vi "Refnum Initialize.vi"(8 "error in (no error)":errorcluster, 11 "QMenu Class in":refnum<class "QMenu Class.lvclass">) -> (0 "error out":errorcluster, 3 "QMenu Class out":refnum<class "QMenu Class.lvclass">)   [LabVIEW 2020, in "QTab.lvlib" / "QMenu Class.lvclass"]
uses:
  QMenu Class.lvclass
  Command Data.ctl
  Command.ctl
  Active Event Data.ctl
  Close Event Data.ctl
  Drag Event Data.ctl
  Image Data.ctl
  <vilib>/picture/picture.llb/imagedata.ctl
  Button Attribute.ctl
  Parameter.ctl
  QMenu Class.lvclass/QMenu Class.ctl
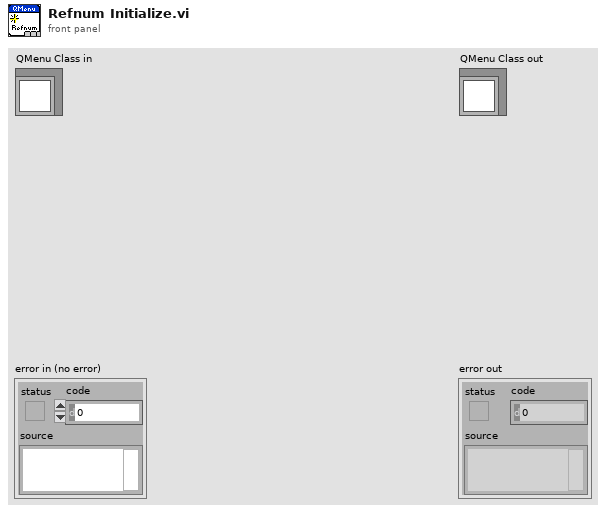
[diagram p1: front panel]
types:
  T1 = typedef "QTab.lvlib/QMenu Class.lvclass/Parameter.ctl" = cluster{"Close Timeout":i32, "Drag Timeout":i32}
  T2 = typedef "QTab.lvlib/QMenu Class.lvclass/Button Attribute.ctl" = cluster{"Label":string, "Button Text":string, "Closable":bool, "Draggable":bool}
  T3 = typedef "QTab.lvlib/QMenu Class.lvclass/Image Data.ctl" = cluster{"Button Image":T4, "Close Button Image":T4, "Left Button Image":T4, "Right Button Image":T4}
  T4 = typedef "imagedata.ctl" = cluster{"image type":i32, "image depth":i32, "image":u8[], "mask":u8[], "colors":u32[], "Rectangle":cluster{"left":i16, "top":i16, "right":i16, "bottom":i16}}
  T5 = typedef "QTab.lvlib/QMenu Class.lvclass/Drag Event Data.ctl" = cluster{"Index":i32, "Label":string, "Vertical":i32, "Horizontal":i32, "Confirm Notifier":refnum<notifier>}
  T6 = typedef "QTab.lvlib/QMenu Class.lvclass/Close Event Data.ctl" = cluster{"Index":i32, "Label":string, "Confirm Notifier":refnum<notifier>}
  T7 = typedef "QTab.lvlib/QMenu Class.lvclass/Active Event Data.ctl" = cluster{"Index":i32, "Label":string}
  T8 = typedef "QTab.lvlib/QMenu Class.lvclass/Command Data.ctl" = cluster{"Command":T9, "Data":variant}
  T9 = typedef "QTab.lvlib/QMenu Class.lvclass/Command.ctl" = enum16{"Initialize", "Get Active Button", "Set Active Button", "Set Button Attribute", "Add Button", "Close Button", "Draw", "Stop"}
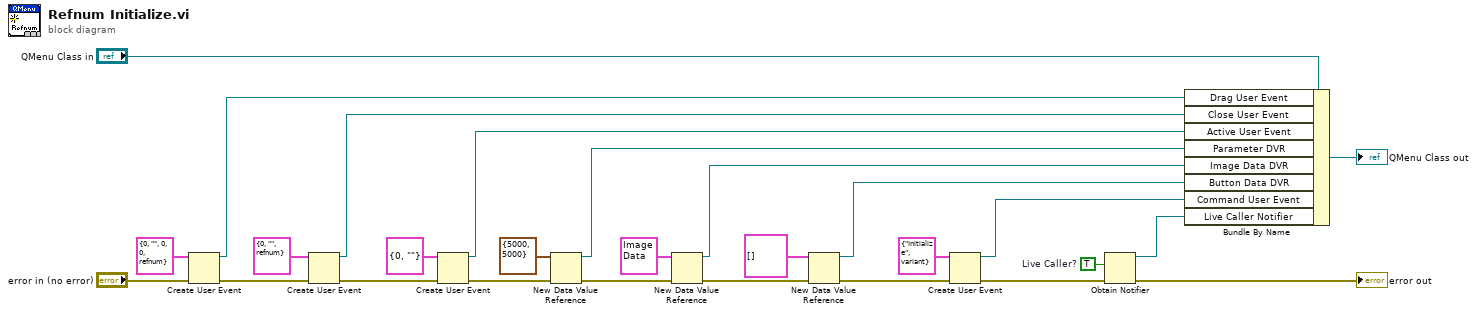
[diagram p0: block diagram]
diagram:
  w23 = TRUE  # Live Caller?
  n1 = Create User Event(user event datatype=T5 {"Index"=0, "Label"="", "Vertical"=0, "Horizontal"=0, "Confirm Notifier"=refnum} ("Drag Event Data"), error in="error in (no error)") -> (user event=w8:refnum<user-event>, error out=w11:errorcluster)
  n2 = Create User Event(user event datatype=T6 {"Index"=0, "Label"="", "Confirm Notifier"=refnum} ("Close Event Data"), error in=w11) -> (user event=w12:refnum<user-event>, error out=w13:errorcluster)
  n3 = Create User Event(user event datatype=T7 {"Index"=0, "Label"=""} ("Active Event Data"), error in=w13) -> (user event=w15:refnum<user-event>, error out=w4:errorcluster)
  n4 = New Data Value Reference(data value=T1 {"Close Timeout"=5000, "Drag Timeout"=5000} ("Parameter"), error in=w4) -> (data value reference=w1:refnum<data-value>, error out=w2:errorcluster)
  n5 = New Data Value Reference(data value=T3 {"Button Image"={"image type"=0, "image depth"=24, "image"=array[19200 elements], "mask"=[], "colors"=[], "Rectangle"={"left"=0, "top"=0, "right"=200, "bottom"=32}}, "Close Button Image"={"image type"=0, "image depth"=32, "image"=[0, 0, 0, 0, 0, 0, 0, 0, 0, 0, 0, 0, 0, 0, 0, 0, 0, 0, 0, 0, 0, 0, 0, 0, 0, 0, 0, 0, 0, 0, 0, 0, 0, 0, 0, 0, 0, 0, 0, 0, 0, 0, 0, 0, 0, 0, 0, 0, 0, 0, 0, 0, 0, 0, 0, 0, 0, 0, 0, 0, 0, 0, 0, 0, 0, 0, 0, 0, 0, 0, 0, 0, 0, 0, 0, 0, 0, 0, 0, 0, 0, 0, 0, 0, 0, 0, 0, 0, 0, 0, 0, 0, 0, 0, 0, 0, 0, 0, 0, 0, 0, 0, 0, 0, 0, 0, 0, 0, 0, 0, 0, 0, 0, 0, 0, 0, 0, 0, 0, 0, 0, 0, 0, 0, 0, 0, 0, 0, 0, 0, 0, 0, 0, 0, 0, 0, 0, 0, 0, 0, 0, 0, 0, 0, 0, 0, 0, 0, 0, 0, 0, 0, 42, 152, 164, 164, 175, 149, 165, 166, 187, 149, 165, 166, 187, 149, 165, 166, 187, 149, 165, 166, 187, 149, 165, 166, 187, 149, 165, 166, 187, 149, 165, 166, 187, 149, 165, 166, 187, 149, 165, 166, 187, 149, 165, 166, 187, 149, 165, 166, 175, 149, 165, 166, 41, 149, 168, 168, 0, 0, 0, 0, 0, 0, 0, 0, 0, 0, 0, 0, 0, 0, 0, 0, 176, 149, 165, 167, 238, 149, 165, 166, 187, 149, 165, 166, 187, 149, 165, 166, 187, 149, 165, 166, 187, 149, 165, 166, 187, 149, 165, 166, 187, 149, 165, 166, 187, 149, 165, 166, 187, 149, 165, 166, 187, 149, 165, 166, 187, 149, 165, 166, 238, 149, 165, 166, 175, 149, 165, 166, 0, 0, 0, 0, 0, 0, 0, 0, 0, 0, 0, 0, 0, 0, 0, 0, 191, 150, 166, 166, 191, 150, 166, 166, 0, 0, 0, 0, 0, 0, 0, 0, 0, 0, 0, 0, 0, 0, 0, 0, 0, 0, 0, 0, 0, 0, 0, 0, 0, 0, 0, 0, 0, 0, 0, 0, 0, 0, 0, 0, 0, 0, 0, 0, 191, 150, 166, 166, 191, 150, 166, 166, 0, 0, 0, 0, 0, 0, 0, 0, 0, 0, 0, 0, 0, 0, 0, 0, 191, 150, 166, 166, 191, 150, 166, 166, 0, 0, 0, 0, 25, 153, 163, 163, 118, 149, 164, 166, 0, 0, 0, 0, 0, 0, 0, 0, 0, 0, 0, 0, 0, 0, 0, 0, 118, 149, 164, 166, 25, 153, 163, 163, 0, 0, 0, 0, 191, 150, 166, 166, 191, 150, 166, 166, 0, 0, 0, 0, 0, 0, 0, 0, 0, 0, 0, 0, 0, 0, 0, 0, 191, 150, 166, 166, 191, 150, 166, 166, 0, 0, 0, 0, 119, 150, 165, 165, 255, 149, 165, 166, 142, 149, 165, 165, 0, 0, 0, 0, 0, 0, 0, 0, 142, 149, 165, 165, 255, 149, 165, 166, 119, 150, 165, 165, 0, 0, 0, 0, 191, 150, 166, 166, 191, 150, 166, 166, 0, 0, 0, 0, 0, 0, 0, 0, 0, 0, 0, 0, 0, 0, 0, 0, 191, 150, 166, 166, 191, 150, 166, 166, 0, 0, 0, 0, 0, 0, 0, 0, 142, 149, 165, 165, 255, 149, 165, 166, 142, 149, 165, 165, 142, 149, 165, 165, 255, 149, 165, 166, 142, 149, 165, 165, 0, 0, 0, 0, 0, 0, 0, 0, 191, 150, 166, 166, 191, 150, 166, 166, 0, 0, 0, 0, 0, 0, 0, 0, 0, 0, 0, 0, 0, 0, 0, 0, 191, 150, 166, 166, 191, 150, 166, 166, 0, 0, 0, 0, 0, 0, 0, 0, 0, 0, 0, 0, 135, 149, 164, 166, 255, 149, 165, 166, 255, 149, 165, 166, 143, 150, 166, 166, 0, 0, 0, 0, 0, 0, 0, 0, 0, 0, 0, 0, 191, 150, 166, 166, 191, 150, 166, 166, 0, 0, 0, 0, 0, 0, 0, 0, 0, 0, 0, 0, 0, 0, 0, 0, 191, 150, 166, 166, 191, 150, 166, 166, 0, 0, 0, 0, 0, 0, 0, 0, 0, 0, 0, 0, 135, 149, 164, 166, 255, 149, 165, 166, 255, 149, 165, 166, 143, 150, 166, 166, 0, 0, 0, 0, 0, 0, 0, 0, 0, 0, 0, 0, 191, 150, 166, 166, 191, 150, 166, 166, 0, 0, 0, 0, 0, 0, 0, 0, 0, 0, 0, 0, 0, 0, 0, 0, 191, 150, 166, 166, 191, 150, 166, 166, 0, 0, 0, 0, 0, 0, 0, 0, 142, 149, 165, 165, 255, 149, 165, 166, 142, 149, 165, 165, 142, 149, 165, 165, 255, 149, 165, 166, 142, 149, 165, 165, 0, 0, 0, 0, 0, 0, 0, 0, 191, 150, 166, 166, 191, 150, 166, 166, 0, 0, 0, 0, 0, 0, 0, 0, 0, 0, 0, 0, 0, 0, 0, 0, 191, 150, 166, 166, 191, 150, 166, 166, 0, 0, 0, 0, 119, 150, 165, 165, 255, 149, 165, 166, 142, 149, 165, 165, 0, 0, 0, 0, 0, 0, 0, 0, 142, 149, 165, 165, 255, 149, 165, 166, 119, 150, 165, 165, 0, 0, 0, 0, 191, 150, 166, 166, 191, 150, 166, 166, 0, 0, 0, 0, 0, 0, 0, 0, 0, 0, 0, 0, 0, 0, 0, 0, 191, 150, 166, 166, 191, 150, 166, 166, 0, 0, 0, 0, 25, 153, 163, 163, 118, 149, 164, 166, 0, 0, 0, 0, 0, 0, 0, 0, 0, 0, 0, 0, 0, 0, 0, 0, 118, 149, 164, 166, 25, 153, 163, 163, 0, 0, 0, 0, 191, 150, 166, 166, 191, 150, 166, 166, 0, 0, 0, 0, 0, 0, 0, 0, 0, 0, 0, 0, 0, 0, 0, 0, 191, 150, 166, 166, 191, 150, 166, 166, 0, 0, 0, 0, 0, 0, 0, 0, 0, 0, 0, 0, 0, 0, 0, 0, 0, 0, 0, 0, 0, 0, 0, 0, 0, 0, 0, 0, 0, 0, 0, 0, 0, 0, 0, 0, 0, 0, 0, 0, 191, 150, 166, 166, 191, 150, 166, 166, 0, 0, 0, 0, 0, 0, 0, 0, 0, 0, 0, 0, 0, 0, 0, 0, 176, 149, 165, 167, 238, 149, 165, 166, 187, 149, 165, 166, 187, 149, 165, 166, 187, 149, 165, 166, 187, 149, 165, 166, 187, 149, 165, 166, 187, 149, 165, 166, 187, 149, 165, 166, 187, 149, 165, 166, 187, 149, 165, 166, 187, 149, 165, 166, 238, 149, 165, 166, 175, 149, 165, 166, 0, 0, 0, 0, 0, 0, 0, 0, 0, 0, 0, 0, 0, 0, 0, 0, 41, 149, 168, 168, 174, 149, 166, 166, 187, 149, 165, 166, 187, 149, 165, 166, 187, 149, 165, 166, 187, 149, 165, 166, 187, 149, 165, 166, 187, 149, 165, 166, 187, 149, 165, 166, 187, 149, 165, 166, 187, 149, 165, 166, 187, 149, 165, 166, 174, 149, 166, 166, 41, 149, 168, 168, 0, 0, 0, 0, 0, 0, 0, 0, 0, 0, 0, 0, 0, 0, 0, 0, 0, 0, 0, 0, 0, 0, 0, 0, 0, 0, 0, 0, 0, 0, 0, 0, 0, 0, 0, 0, 0, 0, 0, 0, 0, 0, 0, 0, 0, 0, 0, 0, 0, 0, 0, 0, 0, 0, 0, 0, 0, 0, 0, 0, 0, 0, 0, 0, 0, 0, 0, 0, 0, 0, 0, 0, 0, 0, 0, 0, 0, 0, 0, 0, 0, 0, 0, 0, 0, 0, 0, 0, 0, 0, 0, 0, 0, 0, 0, 0, 0, 0, 0, 0, 0, 0, 0, 0, 0, 0, 0, 0, 0, 0, 0, 0, 0, 0, 0, 0, 0, 0, 0, 0, 0, 0, 0, 0, 0, 0, 0, 0, 0, 0, 0, 0, 0, 0, 0, 0, 0, 0, 0, 0, 0, 0, 0, 0, 0, 0, 0, 0, 0, 0, 0, 0], "mask"=[0, 0, 0, 0, 0, 0, 0, 0, 31, 254, 0, 0, 63, 255, 0, 0, 48, 3, 0, 0, 48, 3, 0, 0, 51, 51, 0, 0, 51, 243, 0, 0, 49, 227, 0, 0, 49, 227, 0, 0, 51, 243, 0, 0, 51, 51, 0, 0, 48, 3, 0, 0, 48, 3, 0, 0, 63, 255, 0, 0, 31, 254, 0, 0, 0, 0, 0, 0, 0, 0, 0, 0], "colors"=[], "Rectangle"={"left"=0, "top"=0, "right"=18, "bottom"=18}}, "Left Button Image"={"image type"=0, "image depth"=32, "image"=array[2304 elements], "mask"=[0, 0, 0, 0, 0, 0, 0, 0, 0, 0, 0, 0, 15, 255, 240, 0, 31, 255, 248, 0, 24, 0, 24, 0, 24, 0, 24, 0, 24, 4, 24, 0, 24, 14, 24, 0, 24, 28, 24, 0, 24, 56, 24, 0, 24, 112, 24, 0, 24, 112, 24, 0, 24, 56, 24, 0, 24, 28, 24, 0, 24, 14, 24, 0, 24, 4, 24, 0, 24, 0, 24, 0, 24, 0, 24, 0, 31, 255, 248, 0, 15, 255, 240, 0, 0, 0, 0, 0, 0, 0, 0, 0, 0, 0, 0, 0], "colors"=[], "Rectangle"={"left"=0, "top"=4, "right"=24, "bottom"=28}}, "Right Button Image"={"image type"=0, "image depth"=32, "image"=array[2304 elements], "mask"=[0, 0, 0, 0, 0, 0, 0, 0, 0, 0, 0, 0, 15, 255, 240, 0, 31, 255, 248, 0, 24, 0, 24, 0, 24, 0, 24, 0, 24, 32, 24, 0, 24, 112, 24, 0, 24, 56, 24, 0, 24, 28, 24, 0, 24, 14, 24, 0, 24, 14, 24, 0, 24, 28, 24, 0, 24, 56, 24, 0, 24, 112, 24, 0, 24, 32, 24, 0, 24, 0, 24, 0, 24, 0, 24, 0, 31, 255, 248, 0, 15, 255, 240, 0, 0, 0, 0, 0, 0, 0, 0, 0, 0, 0, 0, 0], "colors"=[], "Rectangle"={"left"=0, "top"=4, "right"=24, "bottom"=28}}} ("Image Data"), error in=w2) -> (data value reference=w18:refnum<data-value>, error out=w17:errorcluster)
  n6 = New Data Value Reference(data value=T2[] [] ("Array"), error in=w17) -> (data value reference=w5:refnum<data-value>, error out=w25:errorcluster)
  n7 = Create User Event(user event datatype=T8 {"Command"=enum."Initialize", "Data"=variant} ("Command Data"), error in=w25) -> (user event=w24:refnum<user-event>, error out=w22:errorcluster)
  n8 = Obtain Notifier(notification data type=w23, error in (no error)=w22) -> (notifier out=w19:refnum<notifier>, error out=→"error out":errorcluster)  [unwired: 2 in, 1 out]
  n9 = Bundle By Name(cluster="QMenu Class in", "Drag User Event"=w8, "Close User Event"=w12, "Active User Event"=w15, "Parameter DVR"=w1, "Image Data DVR"=w18, "Button Data DVR"=w5, "Command User Event"=w24, "Live Caller Notifier"=w19) -> (→"QMenu Class out":refnum<class "QMenu Class.lvclass">)
